vi "Sequencer Main.vi"() -> ()   [LabVIEW 2018] (continued)
                  n560 = property on="Sequenser" class="Ring (strict)"("StringsAndValues[]"=w856) -> (error out=w855:errorcluster)  [unwired: 2 in, 1 out]
                  n561 = case shown="True" w843 {
                    tunnel: w850 -> [w866 w870]
                    tunnel: w849 -> [_ w869]
                    tunnel: w847 -> [_ w868]
                    tunnel: [w866 w867] -> w844
                    frame False {
                    }
                    frame True {
                      n562 = Replace Array Subset(array=w870, new element=w868, index=w869) -> (w867:path[])
                    }
                  }
                  n563 = global write "Global Variable.vi" "Sequencer Path"(w844) -> ()
                  n564 = call <userlib>:"Clear All Errors__ogtk.vi"("Error In"=w855) -> ("Error Out"=w854:errorcluster)  [unwired: 3 in]
                }
              }
              n565 = in-place {
                in-place-border: [w819] -> w810
                in-place-border: [w818] -> w809
                in-place-border: w799 -> [w817]
                in-place-border: w798 -> [w816]
                # "Operator"
                n566 = for {
                  N: 5 -> [_]
                  shift-right: [w836] -> w819
                  shift-left: w817 -> [w837]
                  shift-right: [w821] -> w818
                  shift-left: w816 -> [w835]
                  tunnel: [w824] -> _ mode=indexing
                  i -> [w830]
                  n567 = Increment(x=w830) -> (x+1=w826:i32)
                  n568 = Number To Decimal String(number=w826) -> (decimal integer string=w833:string)  [unwired: 1 in]
                  n569 = Concatenate Strings("Name", w833) -> (w832:string)
                  n570 = call-poly <vilib>:"Read Key.vi"("section"="Operator", "error in (no error)"=w835, "key"=w832, "refnum"=w837) -> ("error out"=w823:errorcluster, "value"=w828:string, "refnum out"=w836:T19)  [unwired: 4 in, 1 out]
                  n571 = property on="Operator" class="Ring (strict)"(error in=w823) -> (error out=w822:errorcluster, "StringsAndValues[]"=w825:T33)  [unwired: 1 in, 1 out]
                  n572 = Index Array(array=w825, index=w830) -> (element=w829:cluster{"String":string, "Value":u16})
                  n573 = Bundle By Name(cluster=w829, "String"=w828, "Value"=w826) -> (w827:cluster{"String":string, "Value":u16})
                  n574 = Replace Array Subset(array=w825, new element=w827, index=w826) -> (w824:T33)
                  n575 = property on="Operator" class="Ring (strict)"(error in=w822, "StringsAndValues[]"=w824) -> (error out=w821:errorcluster)  [unwired: 1 in, 1 out]
                }
              }
              n576 = in-place {
                in-place-border: w810 -> [w877]
                in-place-border: w809 -> [w876]
                in-place-border: [w875] -> w808
                in-place-border: [w874] -> w807
                in-place-border: [w873] -> w806
                in-place-border: [w872] -> w805
                in-place-border: [w871] -> w804
                w881 = "REPORT"
                n577 = call-poly <vilib>:"Read Key.vi"("section"=w881, "error in (no error)"=w876, "key"="TOTAL", "refnum"=w877) -> ("error out"=w882:errorcluster, "value"=w873:u32, "refnum out"=w885:T19)  [unwired: 4 in, 1 out]
                n578 = call-poly <vilib>:"Read Key.vi"("section"=w881, "error in (no error)"=w882, "key"="PASS", "refnum"=w885) -> ("error out"=w883:errorcluster, "value"=w872:u32, "refnum out"=w884:T19)  [unwired: 4 in, 1 out]
                n579 = call-poly <vilib>:"Read Key.vi"("section"=w881, "error in (no error)"=w883, "key"="FALSE", "refnum"=w884) -> ("error out"=w874:errorcluster, "value"=w871:u32, "refnum out"=w875:T19)  [unwired: 4 in, 1 out]
              }
              n580 = in-place {
                in-place-border: w808 -> [w887]
                in-place-border: w807 -> [w898]
                # "Read DB Path and Project-Folder create"
                n581 = call-poly <vilib>:"Read Key.vi"("section"="DB", "error in (no error)"=w898, "default value"="D:\\ELETEST_PPROJECTS_DB\\Temp", "key"="Directory", "refnum"=w887) -> ("error out"=w895:errorcluster, "value"=w894:string, "refnum out"=w896:T19)  [unwired: 3 in, 1 out]
                n582 = String To Path(string=w894) -> (path=w886:path)
                n583 = call <vilib>:"Close Config Data.vi"("error in (no error)"=w895, "refnum"=w896) -> ("error out"=w891:errorcluster)  [unwired: 8 in, 1 out]
                n584 = global write "Global Variable.vi" "DB Dir Path"(w886) -> ()
                n585 = call <vilib>:"Check if File or Folder Exists.vi"("error in (no error)"=w891, "path"=w886) -> ("error out"=w888:errorcluster, "file or folder exists?"=w890:bool, "dup path"=w889:path)  [unwired: 7 in]
                n586 = case shown="False" w890 {
                  tunnel: w889 -> [w900 _]
                  tunnel: w888 -> [w899 _]
                  frame False {
                    # "Create Folder"
                    n587 = Create Folder(path (use dialog)=w900, error in=w899) -> ()  [unwired: 1 in, 3 out]
                  }
                  frame True {
                  }
                }
              }
              n588 = local write "Cnt Total All"(w806) -> ()
              n589 = local write "Cnt Pass All"(w805) -> ()
              n590 = local write "Cnt False All"(w804) -> ()
            }
            frame #2 {
              n591 = in-place {
                in-place-border: w905 -> [w993]
                w997 = 0
                w1003 = u32 13816530
                w1004 = u32 0 ("Test Time")
                w982 = bool[] [FALSE, FALSE, FALSE, FALSE, FALSE, FALSE, FALSE, FALSE, FALSE, FALSE] ("Module 0")
                w1007 = 0
                w1019 = T18."Disabled and Grayed Out" ("Disabled")
                w1038 = u32 13816530
                n592 = Bundle(w1038, w1038) -> (w1037:cluster{u32, u32})  [unwired: 1 in]
                n593 = local write "Auto\nRestart"(u16 1 ("Auto\nRestart")) -> ()
                n594 = local write "Cnt Total"(w997) -> ()
                n595 = local write "Cnt Pass"(w997) -> ()
                n596 = local write "Cnt False"(w997) -> ()
                n597 = call <vilib>:"Application Directory.vi"() -> ("Application Directory"=w1033:path)
                n598 = property on="Test Time" class="Str"("Value"="0m - 0s") -> ()  [unwired: 2 in, 2 out]
                n599 = Build Array(w1037) -> (w1036:cluster{u32, u32}[])
                n600 = property on="Tab Control Main" class="TabCtl (strict)"("Value"=T2."INI System" ("Tab Control Main")) -> ()  [unwired: 2 in, 2 out]
                n601 = property on="Dev INI OK?" class="Bool (strict)"("Colors [4]"=w1036, "Value"=TRUE ("Dev INI OK?")) -> ()  [unwired: 2 in, 2 out]
                n602 = property on="Debugging" class="Bool (strict)"("Value"=FALSE ("Debugging")) -> ()  [unwired: 2 in, 2 out]
                n603 = property on="Run Test" class="Bool"("DisabledEnum"=T18."Enabled" ("Disabled")) -> ()  [unwired: 2 in, 2 out]
                n604 = Build Path(base path=w1033, name or relative path="INI\\DeviceConfig.ini") -> (appended path=w1031:path)
                "Device INI Config File Path" <- w1031
                n605 = property on="Tab Control Msg" class="TabCtl (strict)"("Value"=T21."Msg" ("Tab Control Msg")) -> ()  [unwired: 2 in, 2 out]
                n606 = property on="Debug" class="Bool (strict)"("Value"=FALSE) -> ()  [unwired: 2 in, 2 out]
                n607 = property on="Tab Edit/Run" class="TabCtl (strict)"("Value"=enum32{"Edit", "Run"}."Edit" ("Tab Edit/Run")) -> ()  [unwired: 2 in, 2 out]
                n608 = call <vilib>:"Check if File or Folder Exists.vi"("path"=w1031) -> ("error out"=w1032:errorcluster, "file or folder exists?"=w994:bool)  [unwired: 8 in, 1 out]
                n609 = global write "Global Variable.vi" "Current Step Nmb"(w1007) -> ()
                n610 = global write "Global Variable.vi" "Report Step Nmb"(w1007) -> ()
                n611 = global write "Global Variable.vi" "Active Lines Cnt"(w1007) -> ()
                n612 = case shown="True" w994 {
                  tunnel: w1032 -> [w1073 w1078]
                  tunnel: [w1074 w1078] -> w1022
                  frame False {
                    n613 = Bundle By Name(cluster=w1073, "status"=TRUE, "code"=-100, "source"="Ini File not found!") -> (w1074:errorcluster)
                  }
                  frame True {
                  }
                }
                n614 = global write "Global Variable.vi" "Sys ERR"(FALSE ("Sys ERR")) -> ()
                n615 = And(x=w993, y=w994) -> (x .and. y?=→"File Exist?":bool)
                n616 = property on="Button Retest" class="Bool"("DisabledEnum"=w1019) -> ()  [unwired: 2 in, 2 out]
                n617 = property on="Button Next Step" class="Bool"("DisabledEnum"=w1019) -> ()  [unwired: 2 in, 2 out]
                n618 = property on="Break Point Line" class="DigNum (strict)"("DisabledEnum"=w1019) -> ()  [unwired: 2 in, 2 out]
                n619 = global write "Global Variable.vi" "Test Gen Status"(FALSE ("Test Gen Status")) -> ()
                n620 = flat-sequence {
                  frame #0 {
                    n621 = case shown="True" TRUE {
                      frame False {
                      }
                      frame True {
                        n622 = Initialize Array(0.0 ("element"), 100 ("dimension size")) -> (w1050:dbl[])
                        n623 = global write "Global Variable.vi" "Array_Measurement"(w1050) -> ()
                      }
                    }
                  }
                  frame #1 {
                    n624 = case shown="True" TRUE {
                      frame False {
                      }
                      frame True {
                        n625 = global read "Global Variable.vi" "Array_Measurement"() -> (w1059:dbl[])
                        n626 = Replace Array Subset(array=w1059, new element #1=42.15, index #1=1 ("index"), new element #2=10.8, index #2=2 ("index"), new element #3=3.295, index #3=3 ("index")) -> (w1058:dbl[])
                        n627 = global write "Global Variable.vi" "Array_Measurement"(w1058) -> ()
                      }
                    }
                  }
                }
                n628 = global write "Global Variable.vi" "Test Time"(w1004) -> ()
                n629 = global write "Global Variable.vi" "Test Start Time"(w1004) -> ()
                n630 = global write "Global Variable.vi" "Test Stop Time"(w1004) -> ()
                n631 = property on="Serial CMD Mon" class="Str"("Text.Scroll Position"=u32 0, "Value"="") -> ()  [unwired: 2 in, 2 out]
                n632 = call <vilib>:"Open Config Data.vi"("error in (no error)"=w1022, "create file if necessary (T)"=FALSE, "configuration file path"=w1031) -> ("error out"=w1027:errorcluster, "refnum"=w1028:T19)  [unwired: 6 in, 1 out]
                n633 = global read "Global Variable.vi" "Array Errors"() -> (w1024:errorcluster[])
                n634 = Bundle(w1003, w1003) -> (w1002:cluster{u32, u32})  [unwired: 1 in]
                n635 = property on="Msg Str" class="Str"("Value"="") -> ()  [unwired: 2 in, 2 out]
                n636 = call <vilib>:"Get Section Names.vi"("error in (no error)"=w1027, "refnum"=w1028) -> ("error out"=w1030:errorcluster, "section names"=w1026:string[], "refnum out"=w1029:T19)  [unwired: 7 in]
                n637 = Build Array(w1002) -> (w1001:cluster{u32, u32}[])
                n638 = call <vilib>:"Close Config Data.vi"("error in (no error)"=w1030, "refnum"=w1029) -> ()  [unwired: 8 in, 2 out]
                n639 = Replace Array Subset(array=w1024, new element=w1022, index=0) -> (w1023:errorcluster[])
                n640 = property on="Gen Test Status" class="Bool (strict)"("Colors [4]"=w1001, "Value"=TRUE ("Gen Test Status"), "Strings [4]"=string[] ["", "", "", ""]) -> ()  [unwired: 2 in, 2 out]
                n641 = global write "Global Variable.vi" "Dev List"(w1026) -> ()
                n642 = global write "Global Variable.vi" "Array Errors"(w1023) -> ()
                n643 = in-place {
                  # "Set Color of all Row to White (Devices)"
                  n644 = for {
                    N: 15 -> [_]
                    i -> [w1061]
                    n645 = for {
                      N: 8 -> [_]
                      tunnel: w1061 -> [w1065]
                      i -> [w1066]
                      n646 = Bundle By Name(cluster=T15 {"Row"=0, "Column"=0} ("Active Cell:Active Cell"), "Row"=w1065, "Column"=w1066) -> (w1064:T15)
                      n647 = property on="Box Devices" class="MCListbox (strict)"("ActiveCell"=w1064, "CellBG"=u32 16448250) -> ()  [unwired: 2 in, 2 out]
                    }
                  }
                }
                n648 = vi-ref "Sequencer Main.vi"() -> (w991:refnum<vi>)
                n649 = in-place {
                  # "Clear Device Table"
                  n650 = Initialize Array("", 15 ("dimension size"), 8 ("dimension size")) -> (w1070:string[][])
                  n651 = property on="Box Devices" class="MCListbox (strict)"("ItemNames"=w1070, "TopLeft"=T14 {"Row"=0, "Column"=0} ("Top Left Visible Cell")) -> ()  [unwired: 2 in, 2 out]
                }
                n652 = property on="Limits" class="Slide (strict)"("Scale.Maximum"=200.0 ("Data Entry Limits:Maximum"), "Scale.Minimum"=0.0 ("Data Entry Limits:Minimum")) -> ()  [unwired: 2 in, 2 out]
                n653 = global write "Global Variable.vi" "VI Refnum Main"(w991) -> ()
                n654 = call <vilib>:"Application Directory.vi"() -> ("Application Directory"=w989:path)
                n655 = Build Path(base path=w989, name or relative path="INI\\Help.txt") -> (appended path=w990:path)
                n656 = call <vilib>:"Check if File or Folder Exists.vi"("path"=w990) -> ("error out"=w986:errorcluster, "file or folder exists?"=w987:bool, "dup path"=w985:path)  [unwired: 8 in]
                n657 = property on="Help" class="Str"("Value"="Help File Missing") -> (error out=w984:errorcluster)  [unwired: 2 in, 1 out]
                n658 = local read "Switch Relay Modules"() -> (w1009:T5)
                n659 = case shown="True" w987 {
                  tunnel: w986 -> [_ w1046]
                  tunnel: w985 -> [_ w1045]
                  tunnel: w984 -> [_ _]
                  frame False {
                  }
                  frame True {
                    n660 = Open/Create/Replace File(file path (use dialog)=w1045, error in=w1046) -> (refnum out=w1043:refnum<file>, error out=w1044:errorcluster)  [unwired: 4 in, 1 out]
                    n661 = Read from Text File(file (use dialog)=w1043, error in=w1044) -> (refnum out=w1040:refnum<file>, text=w1042:string, error out=w1041:errorcluster)  [unwired: 2 in, 1 out]
                    n662 = local write "Help"(w1042) -> ()
                    n663 = Close File(refnum=w1040, error in=w1041) -> (error out=w1039:errorcluster)  [unwired: 1 out]
                    n664 = call <userlib>:"Clear All Errors__ogtk.vi"("Error In"=w1039) -> ()  [unwired: 3 in, 1 out]
                  }
                }
                n665 = Bundle By Name(cluster=w1009, "SW 0"=w982, "SW 1"=w982, "SW 2"=w982, "SW 3"=w982, "SW 4"=w982, "SW 5"=w982, "SW 6"=w982, "SW 7"=w982) -> (w1010:T5)
                n666 = local write "Switch Relay Modules"(w1010) -> ()
              }
              n667 = for {
                N: 250 -> [_]
                i -> [w908]
                w921 = TRUE ("Active Cell:Cell Font:Bold")
                w919 = T15 {"Row"=0, "Column"=0} ("Active Cell:Active Cell")
                # "PASS/FALSE field"
                # "Set Text Phonts to Test Result collumns"
                n668 = control-ref of="Test Squencer Edit"() -> (w918:refnum<vi>)
                n669 = Bundle By Name(cluster=w919, "Row"=w908, "Column"=5) -> (w940:T15)
                n670 = property on="Property Node" class="MCListbox (strict)"(reference=w918, "ActiveCell"=w940, "CellFontBold"=TRUE ("Active Cell:Cell Font:Bold"), "CellFontSize"=u32 24 ("Active Cell:Cell Font:Size"), "Justify"=enum16{"Left", "Center", "Right"}."Center" ("Active Cell:Cell Justification"), "CellFontColor"=u32 16448250) -> ()  [unwired: 1 in, 2 out]
                n671 = for {
                  N: 3 -> [_]
                  tunnel: w908 -> [w946]
                  tunnel: w919 -> [w945]
                  tunnel: w918 -> [w944]
                  i -> [w943]
                  # "24"
                  n672 = case shown="0, Default" w943 {
                    tunnel: [1 ("Column") 7 8] -> w942
                    tunnel: [u32 20 ("Active Cell:Cell Font:Size") 20 20] -> w941
                    frame 0, Default {
                    }
                    frame 1 {
                    }
                    frame 2 {
                    }
                  }
                  n673 = Bundle By Name(cluster=w945, "Row"=w946, "Column"=w942) -> (w947:T15)
                  n674 = property on="Property Node" class="MCListbox (strict)"(reference=w944, "ActiveCell"=w947, "CellFontSize"=w941) -> ()  [unwired: 1 in, 2 out]
                }
                n675 = control-ref of="Test Sequencer Run"() -> (w922:refnum<vi>)
                n676 = control-ref of="Test Squencer Edit"() -> (w926:refnum<vi>)
                n677 = Bundle By Name(cluster=T15 {"Row"=0, "Column"=0} ("Active Cell:Active Cell"), "Row"=-2, "Column"=-2) -> (w920:T15)
                n678 = property on="Property Node" class="MCListbox (strict)"(reference=w926, "ActiveCell"=w920, "CellFontBold"=w921) -> ()  [unwired: 1 in, 2 out]
                n679 = property on="Property Node" class="MCListbox (strict)"(reference=w922, "ActiveCell"=w920, "CellFontBold"=w921) -> ()  [unwired: 1 in, 2 out]
                n680 = control-ref of="Test Sequencer Run"() -> (w927:refnum<vi>)
                n681 = Bundle By Name(cluster=T15 {"Row"=0, "Column"=0} ("Active Cell:Active Cell"), "Row"=w908, "Column"=5) -> (w928:T15)
                n682 = property on="Property Node" class="MCListbox (strict)"(reference=w927, "ActiveCell"=w928, "CellFontBold"=TRUE ("Active Cell:Cell Font:Bold"), "CellFontSize"=u32 24 ("Active Cell:Cell Font:Size"), "Justify"=enum16{"Left", "Center", "Right"}."Center" ("Active Cell:Cell Justification"), "CellFontColor"=u32 16448250) -> ()  [unwired: 1 in, 2 out]
                n683 = control-ref of="Test Sequencer Run"() -> (w916:refnum<vi>)
                n684 = Bundle By Name(cluster=T15 {"Row"=0, "Column"=0} ("Active Cell:Active Cell"), "Row"=w908, "Column"=1) -> (w915:T15)
                n685 = property on="Property Node" class="MCListbox (strict)"(reference=w916, "ActiveCell"=w915, "CellFontBold"=TRUE ("Active Cell:Cell Font:Bold"), "CellFontSize"=u32 20 ("Active Cell:Cell Font:Size"), "Justify"=enum16{"Left", "Center", "Right"}."Left" ("Active Cell:Cell Justification"), "CellFontColor"=u32 65793) -> ()  [unwired: 1 in, 2 out]
              }
              n686 = in-place {
                # "Set Color of all Row to White"
                n687 = for {
                  N: 250 -> [_]
                  i -> [w969]
                  n688 = for {
                    N: 10 -> [_]
                    tunnel: w969 -> [w974]
                    i -> [w975]
                    n689 = Bundle By Name(cluster=T15 {"Row"=0, "Column"=0} ("Active Cell:Active Cell"), "Row"=w974, "Column"=w975) -> (w973:T15)
                    n690 = property on="Test Squencr Edit" class="MCListbox (strict)"("ActiveCell"=w973, "CellBG"=u32 16448250, "CellFontColor"=u32 0) -> ()  [unwired: 2 in, 2 out]
                  }
                }
              }
              n691 = in-place "In Place Element Structure" {
                # "Cleare Sequencer EDIT Table"
                n692 = Initialize Array("", 250 ("dimension size"), 10 ("dimension size")) -> (w978:string[][])
                n693 = property on="Test Squencr Edit" class="MCListbox (strict)"("ItemNames"=w978, "ActiveCell"=T14 {"Row"=0, "Column"=0} ("Top Left Visible Cell")) -> ()  [unwired: 2 in, 2 out]
              }
              n694 = in-place {
                # "Set Color of all Row RUN Table"
                n695 = for {
                  N: 250 -> [_]
                  i -> [w955]
                  n696 = for {
                    N: 7 -> [_]
                    tunnel: w955 -> [w960]
                    i -> [w961]
                    n697 = Bundle By Name(cluster=T15 {"Row"=0, "Column"=0} ("Active Cell:Active Cell"), "Row"=w960, "Column"=w961) -> (w959:T15)
                    n698 = property on="Test Sequencer Run" class="MCListbox (strict)"("ActiveCell"=w959, "CellBG"=u32 16448250, "CellFontColor"=u32 0) -> ()  [unwired: 2 in, 2 out]
                  }
                }
              }
              n699 = in-place "In Place Element Structure" {
                # "Cleare Sequencer RUN Table"
                n700 = Initialize Array("", 250 ("dimension size"), 7 ("dimension size")) -> (w964:string[][])
                n701 = property on="Test Sequencer Run" class="MCListbox (strict)"("ItemNames"=w964, "ActiveCell"=T14 {"Row"=0, "Column"=0} ("Top Left Visible Cell")) -> ()  [unwired: 2 in, 2 out]
              }
              n702 = in-place {
                n703 = global write "Global Variable.vi" "System Status"(T1."INI Devices" ("System Status")) -> ()
              }
            }
          }
        }
        frame "INI Devices" {
          n704 = flat-sequence {
            frame #0 {
              n705 = in-place {
                # "INI Devices"
                n706 = local read "Device INI Config File Path"() -> (w1080:path)
                n707 = global read "Global Variable.vi" "Dev List"() -> (w1081:string[])
                n708 = Array Size(array=w1081) -> (size(s)=w1082:i32)
                n709 = for {
                  N: w1082 -> [_]
                  tunnel: w1081 -> [w1085] mode=indexing
                  tunnel: w1080 -> [w1084]
                  i -> [w1083]
                  n710 = case shown="\"PICO_SCOPE\"" w1085 {
                    tunnel: w1084 -> [_ w1092 w1104 w1122 w1145 w1149 w1168 w1186]
                    tunnel: w1083 -> [_ w1091 w1105 w1117 w1138 w1148 w1169 w1185]
                    frame "Error", Default {
                      w1087 = u32 16715776
                      n711 = Bundle(w1087, w1087) -> (w1088:cluster{u32, u32})  [unwired: 1 in]
                      n712 = Build Array(w1088) -> (w1089:cluster{u32, u32}[])
                      n713 = property on="Dev INI OK?" class="Bool (strict)"("Colors [4]"=w1089, "Value"=FALSE ("Dev INI OK?")) -> ()  [unwired: 2 in, 2 out]
                      n714 = One Button Dialog(message="Error INI Device File!") -> ()  [unwired: 1 in, 1 out]
                    }
                    frame "DMM_BK5492C" {
                      n715 = control-ref of="Box Devices"() -> (w1093:refnum<vi>)
                      n716 = call "INI_bk5492c.vi"("MCListbox Ref"=w1093, "MListBox Row"=w1091, "Device INI Config File Path"=w1092) -> ("error out"=w1095:errorcluster, "Serial_VISA"=w1094:T34)  [unwired: 7 in]
                      n717 = Unbundle By Name(w1094) -> ("VISA resource name"=w1097:string, "Dev Ok"=w1096:bool)
                      n718 = property on="Dev INI OK?" class="Bool (strict)"() -> ("Value"=w1101:bool)  [unwired: 2 in, 2 out]
                      n719 = global write "Global Variable.vi" "VISA Resource Name BK-5492C"(w1097) -> ()
                      n720 = global read "Global Variable.vi" "Array Errors"() -> (w1100:errorcluster[])
                      n721 = case shown="True" w1101 {
                        tunnel: w1096 -> [_ w1102]
                        frame False {
                        }
                        frame True {
                          n722 = property on="Dev INI OK?" class="Bool (strict)"("Value"=w1102) -> ()  [unwired: 2 in, 2 out]
                        }
                      }
                      n723 = Increment(x=w1091) -> (x+1=w1098:i32)
                      n724 = Replace Array Subset(array=w1100, new element=w1095, index=w1098) -> (w1099:errorcluster[])
                      n725 = global write "Global Variable.vi" "Array Errors"(w1099) -> ()
                    }
                    frame "PS_BK9201" {
                      n726 = control-ref of="Box Devices"() -> (w1107:refnum<vi>)
                      n727 = property on="Dev INI OK?" class="Bool (strict)"() -> ("Value"=w1113:bool)  [unwired: 2 in, 2 out]
                      n728 = call "INI_bk9201.vi"("MCListbox Ref"=w1107, "MCList Box Row"=w1105, "Device INI Config File Path"=w1104) -> ("error out"=w1103:errorcluster, "Serial_VISA"=w1106:T34)  [unwired: 7 in]
                      n729 = Increment(x=w1105) -> (x+1=w1109:i32)
                      n730 = Unbundle By Name(w1106) -> ("VISA resource name"=w1108:string, "Dev Ok"=w1112:bool)
                      n731 = case shown="True" w1113 {
                        tunnel: w1112 -> [_ w1114]
                        frame False {
                        }
                        frame True {
                          n732 = property on="Dev INI OK?" class="Bool (strict)"("Value"=w1114) -> ()  [unwired: 2 in, 2 out]
                        }
                      }
                      n733 = global write "Global Variable.vi" "VISA Resource Name BK-9202"(w1108) -> ()
                      n734 = global read "Global Variable.vi" "Array Errors"() -> (w1111:errorcluster[])
                      n735 = Replace Array Subset(array=w1111, new element=w1103, index=w1109) -> (w1110:errorcluster[])
                      n736 = global write "Global Variable.vi" "Array Errors"(w1110) -> ()
                    }
                    frame "FTDI_SPI_Sys" {
                      # "100000"
                      n737 = control-ref of="Box Devices"() -> (w1120:refnum<vi>)
                      n738 = property on="Dev INI OK?" class="Bool (strict)"() -> ("Value"=w1126:bool)  [unwired: 2 in, 2 out]
                      n739 = call "INI_SPI_Sysl.vi"("MCListbox Ref"=w1120, "MListBox Row"=w1117, "config"=T22 {"ClockRate"=1000, "LatencyTimer"=10, "configOptions 24-31"=0, "configOptions 16-23"=0, "configOptions 8-15"=0, "configOptions 0-7"=32, "Pin"=0, "reserved"=0}, "Device INI Config File Path"=w1122) -> ("error out"=w1118:errorcluster, "Dev OK"=w1119:bool, "Handle"=w1116:u32)  [unwired: 5 in]
                      n740 = case shown="True" w1126 {
                        tunnel: w1119 -> [_ w1134]
                        frame False {
                        }
                        frame True {
                          n741 = property on="Dev INI OK?" class="Bool (strict)"("Value"=w1134) -> ()  [unwired: 2 in, 2 out]
                        }
                      }
                      n742 = global read "Global Variable.vi" "Array Errors"() -> (w1125:errorcluster[])
                      n743 = global write "Global Variable.vi" "FTDI SPI Handle"(w1116) -> ()
                      n744 = Increment(x=w1117) -> (x+1=w1123:i32)
                      n745 = Replace Array Subset(array=w1125, new element=w1118, index=w1123) -> (w1124:errorcluster[])
                      n746 = global write "Global Variable.vi" "Array Errors"(w1124) -> ()
                      n747 = for {
                        N: 8 -> [_]
                        tunnel: w1116 -> [w1128]
                        i -> [w1129]
                        w1131 = u8 0  # nCS
                        w1130 = u16 0  # Channel Decimal
                        w1132 = TRUE  # Use Extra
                        # "RESET ALL Relay"
                        n748 = call "FTDI SPI GPIO Set.vi"("nCS"=w1131, "Mode"=T23."Set Decimal", "Use Extra"=w1132, "Channel Decimal"=w1130, "Addr"=w1129, "Handler In"=w1128) -> ("error out"=w1127:errorcluster)  [unwired: 2 in, 3 out]
                        n749 = call <userlib>:"Clear All Errors__ogtk.vi"("Upsteam Error (optional)"=w1127, "Error In"=w1127) -> ()  [unwired: 2 in, 1 out]
                      }
                    }
                    frame "FTDI_RS232_App" {
                      n750 = control-ref of="Box Devices"() -> (w1144:refnum<vi>)
                      n751 = property on="Dev INI OK?" class="Bool (strict)"() -> ("Value"=w1142:bool)  [unwired: 2 in, 2 out]
                      n752 = Increment(x=w1138) -> (x+1=w1137:i32)
                      n753 = call "INI_RS232_Appl.vi"("Device INI Config File Path"=w1145, "MListBox Row"=w1138, "MCListbox Ref"=w1144) -> ("COM Port"=w1135:refnum<visa-resource-name>, "Dev OK"=w1141:bool, "Handle"=w1143:u32, "error out"=w1136:errorcluster)  [unwired: 4 in]
                      n754 = case shown="True" w1142 {
                        tunnel: w1141 -> [_ w1146]
                        frame False {
                        }
                        frame True {
                          n755 = property on="Dev INI OK?" class="Bool (strict)"("Value"=w1146) -> ()  [unwired: 2 in, 2 out]
                        }
                      }
                      n756 = global write "Global Variable.vi" "COM Port FTDI RS232"(w1135) -> ()
                      n757 = global write "Global Variable.vi" "FTDI RS232 Handle"(w1143) -> ()
                      n758 = global read "Global Variable.vi" "Array Errors"() -> (w1140:errorcluster[])
                      n759 = Replace Array Subset(array=w1140, new element=w1136, index=w1137) -> (w1139:errorcluster[])
                      n760 = global write "Global Variable.vi" "Array Errors"(w1139) -> ()
                    }
                    frame "PICO_SCOPE" {
                      n761 = flat-sequence {
                        tunnel: w1149 -> [w1152]
                        tunnel: [w1152] -> w1147
                        tunnel: w1148 -> [w1158]
                        tunnel: w1147 -> [w1163]
                        frame #0 {
                          n762 = global read "Global Variable.vi" "PicoScope Handle"() -> (w1150:u32)
                          n763 = Greater Than 0?(x=w1150) -> (x > 0?=w1151:bool)
                          n764 = case shown="True" w1151 {
                            tunnel: w1150 -> [_ w1153]
                            frame False {
                            }
                            frame True {
                              n765 = call "PicoScope3000aClose.vi"("handle"=w1153) -> ()
                            }
                          }
                        }
                        frame #1 {
                          n766 = control-ref of="Box Devices"() -> (w1162:refnum<vi>)
                          n767 = property on="Dev INI OK?" class="Bool (strict)"() -> ("Value"=w1166:bool)  [unwired: 2 in, 2 out]
                          n768 = call "INI_PicoScope.vi"("MCListbox Ref"=w1162, "MListBox Row"=w1158, "Device INI Config File Path"=w1163) -> ("error out"=w1160:errorcluster, "Handle"=w1159:u32, "Dev OK"=w1161:bool, "Device Info"=w1154:T35, "Max Adc value"=w1157:i16, "PicoScope Correction"=w1155:i32)  [unwired: 2 in]
                          n769 = case shown="True" w1166 {
                            tunnel: w1161 -> [_ w1167]
                            frame False {
                            }
                            frame True {
                              n770 = property on="Dev INI OK?" class="Bool (strict)"("Value"=w1167) -> ()  [unwired: 2 in, 2 out]
                            }
                          }
                          n771 = global write "Global Variable.vi" "PicoScope Device Info"(w1154) -> ()
                          n772 = global read "Global Variable.vi" "Array Errors"() -> (w1165:errorcluster[])
                          n773 = global write "Global Variable.vi" "PicoScope Correction"(w1155) -> ()
                          n774 = global write "Global Variable.vi" "PicoScope Handle"(w1159) -> ()
                          n775 = global write "Global Variable.vi" "PicoScope Max Adc Value"(w1157) -> ()
                          n776 = Increment(x=w1158) -> (x+1=w1156:i32)
                          n777 = Replace Array Subset(array=w1165, new element=w1160, index=w1156) -> (w1164:errorcluster[])
                          n778 = global write "Global Variable.vi" "Array Errors"(w1164) -> ()
                        }
                      }
                    }
                    frame "BLE" {
                      n779 = control-ref of="Box Devices"() -> (w1175:refnum<vi>)
                      n780 = Increment(x=w1169) -> (x+1=w1171:i32)
                      n781 = call "INI_BLE.vi"("MCListbox Ref"=w1175, "MListBox Row"=w1169, "Device INI Config File Path"=w1168) -> ("error out"=w1172:errorcluster, "ComPort"=w1170:refnum<visa-resource-name>)  [unwired: 5 in, 1 out]
                      n782 = global write "Global Variable.vi" "COM Port BLE"(w1170) -> ()
                      n783 = global read "Global Variable.vi" "Array Errors"() -> (w1174:errorcluster[])
                      n784 = Replace Array Subset(array=w1174, new element=w1172, index=w1171) -> (w1173:errorcluster[])
                      n785 = global write "Global Variable.vi" "Array Errors"(w1173) -> ()
                    }
                    frame "FTDI_RS232_RFID" {
                      n786 = control-ref of="Box Devices"() -> (w1184:refnum<vi>)
                      n787 = Increment(x=w1185) -> (x+1=w1187:i32)
                      n788 = call "INI_RS232_RFID.vi"("Device INI Config File Path"=w1186, "MListBox Row"=w1185, "MCListbox Ref"=w1184) -> ("RFID Power"=w1183:u16, "COM Port"=w1182:refnum<visa-resource-name>, "Dev OK"=w1177:bool, "Handle"=w1178:u32, "error out"=w1179:errorcluster)  [unwired: 3 in]
                      n789 = global write "Global Variable.vi" "FTDI RS232 Handle  RFID"(w1178) -> ()
                      n790 = global write "Global Variable.vi" "COM Port RFID"(w1182) -> ()
                      n791 = case shown="False" FALSE {
                        tunnel: w1179 -> [w1191 w1196]
                        tunnel: w1183 -> [_ w1194]
                        tunnel: w1182 -> [_ w1195]
                        tunnel: [w1191 w1192] -> w1181
                        tunnel: [FALSE w1193] -> _
                        frame False {
                        }
                        frame True {
                          n792 = call <userlib>:"Clear All Errors__ogtk.vi"("Error In"=w1196) -> ()  [unwired: 3 in, 1 out]
                          n793 = global write "Global Variable.vi" "RFID Power"(w1194) -> ()
                          n794 = call "Ini RFID ftdi.vi"("Power"=w1194, "COM RFID"=w1195) -> ("Err Out"=w1192:errorcluster, "Ini ?"=w1193:bool)  [unwired: 7 in, 1 out]
                        }
                      }
                      n795 = global read "Global Variable.vi" "Array Errors"() -> (w1189:errorcluster[])
                      n796 = property on="Dev INI OK?" class="Bool (strict)"() -> ("Value"=w1180:bool)  [unwired: 2 in, 2 out]
                      n797 = Replace Array Subset(array=w1189, new element=w1181, index=w1187) -> (w1188:errorcluster[])
                      n798 = case shown="True" w1180 {
                        tunnel: w1177 -> [_ w1197]
                        frame False {
                        }
                        frame True {
                          n799 = property on="Dev INI OK?" class="Bool (strict)"("Value"=w1197) -> ()  [unwired: 2 in, 2 out]
                        }
                      }
                      n800 = global write "Global Variable.vi" "Array Errors"(w1188) -> ()
                    }
                  }
                }
              }
            }
            frame #1 {
              n801 = property on="Dev INI OK?" class="Bool (strict)"() -> ("Value"=w1203:bool)  [unwired: 2 in, 2 out]
              n802 = for {
                N: 8 -> [_]
                i -> [w1205]
                # "Reset Relay Leds Indicator"
                n803 = case shown="6" w1205 {
                  tunnel: bool[] [] ("Boolean array") -> [_ w1207 w1210 w1213 w1216 w1219 w1222 w1225]
                  frame -1, Default {
                  }
                  frame 0 {
                    n804 = local read "Switch Relay Modules"() -> (w1209:T5)
                    n805 = Bundle By Name(cluster=w1209, "SW 0"=w1207) -> (w1208:T5)
                    n806 = local write "Switch Relay Modules"(w1208) -> ()
                  }
                  frame 1 {
                    n807 = local read "Switch Relay Modules"() -> (w1212:T5)
                    n808 = Bundle By Name(cluster=w1212, "SW 1"=w1210) -> (w1211:T5)
                    n809 = local write "Switch Relay Modules"(w1211) -> ()
                  }
                  frame 2 {
                    n810 = local read "Switch Relay Modules"() -> (w1215:T5)
                    n811 = Bundle By Name(cluster=w1215, "SW 2"=w1213) -> (w1214:T5)
                    n812 = local write "Switch Relay Modules"(w1214) -> ()
                  }
                  frame 3 {
                    n813 = local read "Switch Relay Modules"() -> (w1218:T5)
                    n814 = Bundle By Name(cluster=w1218, "SW 3"=w1216) -> (w1217:T5)
                    n815 = local write "Switch Relay Modules"(w1217) -> ()
                  }
                  frame 4 {
                    n816 = local read "Switch Relay Modules"() -> (w1221:T5)
                    n817 = Bundle By Name(cluster=w1221, "SW 4"=w1219) -> (w1220:T5)
                    n818 = local write "Switch Relay Modules"(w1220) -> ()
                  }
                  frame 5 {
                    n819 = local read "Switch Relay Modules"() -> (w1224:T5)
                    n820 = Bundle By Name(cluster=w1224, "SW 5"=w1222) -> (w1223:T5)
                    n821 = local write "Switch Relay Modules"(w1223) -> ()
                  }
                  frame 6 {
                    n822 = local read "Switch Relay Modules"() -> (w1227:T5)
                    n823 = Bundle By Name(cluster=w1227, "SW 6"=w1225) -> (w1226:T5)
                    n824 = local write "Switch Relay Modules"(w1226) -> ()
                  }
                }
              }
              n825 = case shown="False" "Debug" {
                tunnel: [w1228 w1230] -> w1204
                tunnel: w1203 -> [w1228 w1229]
                frame False {
                }
                frame True {
                  n826 = Not(x=w1229) -> (.not. x?=w1230:bool)
                }
              }
              n827 = global read "Global Variable.vi" "PicoScope Correction"() -> (w1200:i32)
              n828 = case shown="False" w1204 {
                frame False {
                  w1232 = u32 16715776
                  n829 = Bundle(w1232, w1232) -> (w1234:cluster{u32, u32})  [unwired: 1 in]
                  n830 = Build Array(w1234) -> (w1233:cluster{u32, u32}[])
                  n831 = property on="Dev INI OK?" class="Bool (strict)"("Colors [4]"=w1233, "Value"=FALSE ("Dev INI OK?")) -> ()  [unwired: 2 in, 2 out]
                }
                frame True {
                  w1237 = u32 6618880
                  n832 = Bundle(w1237, w1237) -> (w1236:cluster{u32, u32})  [unwired: 1 in]
                  n833 = Build Array(w1236) -> (w1235:cluster{u32, u32}[])
                  n834 = property on="Dev INI OK?" class="Bool (strict)"("Colors [4]"=w1235, "Value"=FALSE ("Dev INI OK?")) -> ()  [unwired: 2 in, 2 out]
                }
              }
              n835 = Add(x=290, y=w1200) -> (x+y=w1199:i32)
              n836 = local write "Pico Scope Correction"(w1199) -> ()
            }
          }
          n837 = in-place {
            n838 = global write "Global Variable.vi" "System Status"(T1."Idle" ("System Status")) -> ()
          }
        }
        frame "INI Secuencer" {
          n839 = flat-sequence {
            tunnel: [w1241] -> w1240
            tunnel: w1240 -> [w1250]
            tunnel: [w1250] -> w1239
            tunnel: w1239 -> [w1360]
            frame #0 {
              n840 = local read "Barcode\nDefault"() -> (w1243:bool)
              n841 = global read "Global Variable.vi" "Customer"() -> (w1245:string)
              n842 = global read "Global Variable.vi" "Config"() -> (w1246:string)
              n843 = global read "Global Variable.vi" "Board"() -> (w1244:string)
              n844 = property on="Test Squencer Edit" class="MCListbox (strict)"("Visible"=TRUE) -> ()  [unwired: 2 in, 2 out]
              n845 = case shown="True" w1243 {
                frame False {
                  n846 = property on="Barcode" class="Str"("Value"="", "Key Focus"=TRUE) -> ()  [unwired: 2 in, 2 out]
                }
                frame True {
                  n847 = property on="Barcode" class="Str"("Value"="ADB-12345") -> ()  [unwired: 2 in, 2 out]
                }
              }
              n848 = local write "Under Test BOARD"(w1244) -> ()
              n849 = local write "Customer"(w1245) -> ()
              n850 = local write "Config"(w1246) -> ()
              n851 = call <vilib>:"Set Busy.vi"() -> ("error out"=w1241:errorcluster)  [unwired: 10 in, 1 out]
            }
            frame #1 {
              n852 = global read "Sequencer Array.vi" "SEQUENCER Array"() -> (w1251:T16[])
              n853 = Array Size(array=w1251) -> (size(s)=w1252:i32)
              n854 = for {
                N: w1252 -> [_]
                tunnel: w1251 -> [w1263] mode=indexing
                i -> [w1253]
                # "Revrite Table"
                n855 = Unbundle By Name(w1263) -> ("Step Type"=w1258:u16, "Step Description"=w1280:string, "Test Values.Str Value"=w1276:string, "Test Result"=w1275:T17, "Measure Units"=w1273:string, "Parameters"=w1270:string, "Step ID"=w1271:u16, "Test Values.Numeric Value"=w1278:dbl, "Test Values.Upper Limit"=w1269:dbl, "Test Values.Lower Limit"=w1268:dbl, "Run/Skip"=w1262:bool, "Report"=w1267:bool)  [unwired: 1 out]
                n856 = case shown="0, Default" w1258 {
                  tunnel: ["- (Label)" "- (Sets)" "- (Numb)" "- (String)" "- (Bool)"] -> w1282
                  tunnel: [FALSE FALSE TRUE FALSE FALSE] -> w1279
                  frame 0, Default {
                  }
                  frame 1 {
                  }
                  frame 2 {
                  }
                  frame 3 {
                  }
                  frame 4 {
                  }
                }
                n857 = case shown="False" w1267 {
                  tunnel: ["No" "Yes"] -> w1265
                  frame False {
                  }
                  frame True {
                  }
                }
                n858 = case shown="True" w1262 {
                  tunnel: ["Skip" "Run"] -> w1266
                  frame False {
                  }
                  frame True {
                  }
                }
                n859 = Number To Decimal String(number=w1271) -> (decimal integer string=w1264:string)  [unwired: 1 in]
                n860 = case shown="\"Idle\", Default" w1275 {
                  tunnel: ["Idle" "PASS" "FALSE"] -> w1274
                  frame "Idle", Default {
                  }
                  frame "PASS" {
                  }
                  frame "FALSE" {
                  }
                }
                n861 = Number To Decimal String(number=w1253) -> (decimal integer string=w1283:string)  [unwired: 1 in]
                n862 = case shown="True" w1279 {
                  tunnel: [w1333 w1342] -> w1272
                  tunnel: [w1333 w1339] -> w1277
                  tunnel: w1278 -> [_ w1337]
                  tunnel: w1269 -> [_ w1336]
                  tunnel: w1268 -> [_ w1335]
                  tunnel: w1273 -> [_ w1334]
                  frame False {
                    w1333 = "..."
                  }
                  frame True {
                    n863 = Format Into String(format string="max %5.2f", w1336) -> (resulting string=w1344:string)  [unwired: 2 in, 1 out]
                    n864 = Format Into String(format string="min %5.2f", w1335) -> (resulting string=w1343:string)  [unwired: 2 in, 1 out]
                    n865 = Format Into String(format string="%5.2f", w1337) -> (resulting string=w1341:string)  [unwired: 2 in, 1 out]
                    n866 = Concatenate Strings(w1344, "\r", w1343) -> (w1342:string)
                    n867 = Concatenate Strings(w1341, " (", w1334, ")") -> (w1339:string)
                  }
                }
                n868 = Concatenate Strings(w1283, w1282) -> (w1281:string)
                n869 = property on="Test Squencr Edit" class="MCListbox (strict)"() -> ("ItemNames"=w1260:string[][])  [unwired: 2 in, 2 out]
                n870 = Build Array(w1281, w1280, w1277, w1276, w1272, w1274, w1266, w1270, w1264, w1265) -> (w1261:string[])
                n871 = Replace Array Subset(array=w1260, new element=w1261, index (row)=w1253) -> (w1259:string[][])  [unwired: 1 in]
                n872 = Bundle By Name(cluster=T15 {"Row"=0, "Column"=0} ("Active Cell:Active Cell"), "Row"=w1253, "Column"=5) -> (w1257:T15)
                n873 = property on="Test Squencr Edit" class="MCListbox (strict)"("ItemNames"=w1259, "Value"=w1253, "ActiveCell"=w1257, "CellFontColor"=u32 16448250) -> ()  [unwired: 2 in, 2 out]
                n874 = in-place {
                  in-place-border: w1253 -> [w1284]
                  n875 = Quotient & Remainder(x=w1284, y=20) -> (x-y*floor(x/y)=w1288:i32)  [unwired: 1 out]
                  n876 = Increment(x=w1284) -> (x+1=w1285:i32)
                  n877 = Equal?(x=w1288, y=u32 0) -> (x = y?=w1286:bool)
                  n878 = case shown="True" w1286 {
                    tunnel: w1285 -> [_ w1290]
                    frame False {
                    }
                    frame True {
                      n879 = Bundle By Name(cluster=T14 {"Row"=0, "Column"=0} ("Top Left Visible Cell"), "Row"=w1290) -> (w1291:T14)
                      n880 = property on="Test Sequencer" class="MCListbox (strict)"("TopLeft"=w1291) -> ()  [unwired: 2 in, 2 out]
                    }
                  }
                }
                n881 = in-place {
                  in-place-border: w1262 -> [w1295]
                  in-place-border: w1258 -> [w1294]
                  in-place-border: w1253 -> [w1293]
                  n882 = case shown="True" w1295 {
                    tunnel: w1293 -> [w1296 w1303]
                    tunnel: w1294 -> [_ w1304]
                    frame False {
                      n883 = for {
                        N: 8 -> [_]
                        tunnel: w1296 -> [w1300]
                        i -> [w1301]
                        n884 = Bundle By Name(cluster=T15 {"Row"=0, "Column"=0} ("Active Cell:Active Cell"), "Row"=w1300, "Column"=w1301) -> (w1299:T15)
                        n885 = property on="Test Sequencer" class="MCListbox (strict)"("ActiveCell"=w1299, "CellBG"=u32 14606046) -> ()  [unwired: 2 in, 2 out]
                      }
                    }
                    frame True {
                      n886 = case shown="1" w1304 {
                        tunnel: w1303 -> [w1305 w1312 w1319]
                        frame 999, Default {
                          n887 = for {
                            N: 10 -> [_]
                            tunnel: w1305 -> [w1309]
                            i -> [w1310]
                            n888 = Bundle By Name(cluster=T15 {"Row"=0, "Column"=0} ("Active Cell:Active Cell"), "Row"=w1309, "Column"=w1310) -> (w1308:T15)
                            n889 = property on="Test Sequencer" class="MCListbox (strict)"("ActiveCell"=w1308, "CellBG"=u32 16448250) -> ()  [unwired: 2 in, 2 out]
                          }
                        }
                        frame 0 {
                          n890 = for {
                            N: 10 -> [_]
                            tunnel: w1312 -> [w1316]
                            i -> [w1317]
                            n891 = Bundle By Name(cluster=T15 {"Row"=0, "Column"=0} ("Active Cell:Active Cell"), "Row"=w1316, "Column"=w1317) -> (w1315:T15)
                            n892 = property on="Test Sequencer" class="MCListbox (strict)"("ActiveCell"=w1315, "CellBG"=u32 16772930) -> ()  [unwired: 2 in, 2 out]
                          }
                        }
                        frame 1 {
                          n893 = for {
                            N: 10 -> [_]
                            tunnel: w1319 -> [w1323]
                            i -> [w1324]
                            n894 = Bundle By Name(cluster=T15 {"Row"=0, "Column"=0} ("Active Cell:Active Cell"), "Row"=w1323, "Column"=w1324) -> (w1322:T15)
                            n895 = property on="Test Sequencer" class="MCListbox (strict)"("ActiveCell"=w1322, "CellBG"=u32 13627391) -> ()  [unwired: 2 in, 2 out]
                          }
                        }
                      }
                    }
                  }
                }
              }
            }
            frame #2 {
              n896 = call <vilib>:"Unset Busy.vi"("error in (no error)"=w1360) -> ("error out"=w1359:errorcluster)  [unwired: 10 in]
              n897 = call <userlib>:"Clear All Errors__ogtk.vi"("Error In"=w1359) -> ()  [unwired: 3 in, 1 out]
              n898 = property on="Test Sequencer" class="MCListbox (strict)"("TopLeft"=T14 {"Row"=0, "Column"=0} ("Top Left Visible Cell"), "Value"=T11 0 ("Test Squencer Edit")) -> ()  [unwired: 2 in, 2 out]
              n899 = property on="Test Squencer Edit" class="MCListbox (strict)"("Visible"=TRUE) -> ()  [unwired: 2 in, 2 out]
              n900 = global write "Global Variable.vi" "Reset BARCODE"(TRUE ("Reset BARCODE")) -> ()
            }
            frame #3 {
              n901 = in-place {
                n902 = global write "Global Variable.vi" "System Status"(T1."Idle" ("System Status")) -> ()
              }
            }
          }
        }
        frame "START Sequencer" {
          n903 = flat-sequence {
            tunnel: [w1376] -> w1369
            tunnel: [w1375] -> w1368
            tunnel: w1367 -> [w1370]
            tunnel: w1366 -> [w1371]
            tunnel: w1369 -> [_]
            tunnel: w1368 -> [_]
            frame #0 {
              w1373 = FALSE ("Auto\nReStart")
              w1372 = u16 0 ("Gen Err Cnt")
              n904 = in-place {
                in-place-border: w1371 -> [w1383]
                in-place-border: w1370 -> [w1382]
                # "Set SYS-Out Relay"
                n905 = call <vilib>:"Acquire Semaphore.vi"("error in (no error)"=w1383, "semaphore"=w1382) -> ("error out"=w1380:errorcluster, "semaphore out"=w1381:T13)  [unwired: 3 in, 1 out]
                n906 = case shown="No Error" w1380 {
                  selector: w1380 -> [w1387 w1400]
                  tunnel: w1381 -> [w1390 w1399]
                  tunnel: [w1389 w1400] -> w1379
                  tunnel: [w1388 w1399] -> w1378
                  frame No Error {
                    n907 = in-place {
                      in-place-border: [w1393] -> w1389
                      in-place-border: w1387 -> [w1393]
                      in-place-border: [w1392] -> w1388
                      in-place-border: w1390 -> [w1392]
                      w1396 = T20 7 items=["Addr-0"=0, "Addr-1"=4, "Addr-2"=2, "Addr-3"=6, "Addr-4"=1, "Addr-5"=5, "Addr-6"=3, "Addr-7"=7] ("Addr")
                      n908 = global read "Global Variable.vi" "FTDI SPI Handle"() -> (w1398:u32)
                      n909 = call "FTDI SPI GPIO Set.vi"("nCS"=u8 2, "Mode"=T24."Set Decimal", "Use Extra"=TRUE, "Channel Decimal"=u16 0, "Addr"=w1396, "Handler In"=w1398) -> ()  [unwired: 2 in, 4 out]
                    }
                    n910 = local read "Switch Relay Modules"() -> (w1386:T5)
                    n911 = Bundle By Name(cluster=w1386, "SW 7"=bool[] [FALSE, FALSE, FALSE, FALSE, FALSE, FALSE, FALSE, FALSE]) -> (w1385:T5)
                    n912 = local write "Switch Relay Modules"(w1385) -> ()
                  }
                  frame Error {
                  }
                }
                n913 = call <vilib>:"Release Semaphore.vi"("error in (no error)"=w1379, "semaphore"=w1378) -> ()  [unwired: 4 in, 2 out]
              }
              n914 = in-place {
                w1403 = u32 12369084
                n915 = Tick Count (ms)() -> (millisecond timer value=w1409:u32)
                n916 = global write "Global Variable.vi" "Test Stop Time"(w1409) -> ()
                n917 = global write "Global Variable.vi" "Test Start Time"(w1409) -> ()
                n918 = global write "Global Variable.vi" "Test Time"(u32 0 ("Test Start Time")) -> ()
                n919 = property on="Test Time" class="Str"("Value"="0m - 0s") -> ()  [unwired: 2 in, 2 out]
                n920 = Bundle(w1403, w1403) -> (w1404:cluster{u32, u32})  [unwired: 1 in]
                n921 = Build Array(w1404) -> (w1405:cluster{u32, u32}[])
                n922 = global write "Global Variable.vi" "Test Gen Status"(TRUE ("Test Gen Status")) -> ()
                n923 = property on="Gen Test Status" class="Bool (strict)"("Colors [4]"=w1405, "Value"=TRUE ("Gen Test Status"), "Strings [4]"=string[] ["", "", "", ""]) -> ()  [unwired: 2 in, 2 out]
              }
              n924 = global write "Global Variable.vi" "Gen Err Cnt"(w1372) -> ()
              n925 = global write "Global Variable.vi" "Active Lines Cnt"(w1372) -> ()
              n926 = global write "Global Variable.vi" "Retest Cnt"(w1372) -> ()
              n927 = global write "Global Variable.vi" "Cancel by operator"(w1373) -> ()
              n928 = global write "Global Variable.vi" "Retest ON"(w1373) -> ()
              n929 = local write "Auto\nReStart"(w1373) -> ()
              n930 = property on="Dev INI OK?" class="Bool (strict)"("Value"=TRUE ("Dev INI OK?")) -> (error out=w1376:errorcluster)  [unwired: 2 in, 1 out]
              n931 = property on="Msg Str" class="Str"("Value"="START SEQUENCER INI") -> (error out=w1375:errorcluster)  [unwired: 2 in, 1 out]
            }
            frame #1 {
              n932 = local read "Auto\nRestart"() -> (w1412:u16)
              n933 = local read "Restart Cnt"() -> (w1411:u16)
              n934 = Less?(x=w1411, y=w1412) -> (x < y?=w1410:bool)
              n935 = case shown="True" w1410 {
                frame False {
                }
                frame True {
                  n936 = local read "Restart Cnt"() -> (w1414:u16)
                  n937 = Increment(x=w1414) -> (x+1=w1413:u16)
                  n938 = local write "Restart Cnt"(w1413) -> ()
                }
              }
            }
            frame #2 {
              n939 = local read "Barcode\nDefault"() -> (w1416:bool)
              n940 = case shown="True" w1416 {
                tunnel: [w1417 w1418] -> w1415
                frame False {
                  n941 = property on="Barcode" class="Str"() -> ("Value"=w1417:string)  [unwired: 2 in, 2 out]
                }
                frame True {
                  n942 = local read "Auto\nRestart"() -> (w1420:u16)
                  n943 = Greater?(x=w1420, y=1) -> (0:w1419:bool)
                  n944 = case shown="False" w1419 {
                    tunnel: ["ADB-12345" w1423] -> w1418
                    frame False {
                    }
                    frame True {
                      n945 = local read "Restart Cnt"() -> (w1431:u16)
                      n946 = Number To Decimal String(number=w1431) -> (decimal integer string=w1425:string)  [unwired: 1 in]
                      n947 = String Length(string=w1425) -> (length=w1428:i32)
                      n948 = Subtract(x=5, y=w1428) -> (x-y=w1426:i32)
                      n949 = Replace Substring(3:w1426, 4:w1425, 5:"00000") -> (1:w1424:string)  [unwired: 1 in, 1 out]
                      n950 = Concatenate Strings("ADB-", w1424) -> (w1423:string)
                    }
                  }
                  n951 = property on="Barcode" class="Str"("Value"=w1418) -> ()  [unwired: 2 in, 2 out]
                }
              }
              n952 = global write "Global Variable.vi" "Baccode MEM"(w1415) -> ()
            }
            frame #3 {
